vi "PKG_IMC_MoveAbs.vi"(4 "axis":i32, 5 "wait":i32, 6 "tgvel":dbl, 7 "endvel":dbl, 9 "startvel":dbl, 10 "pos":i32, 11 "handle":u32) -> (2 "function return":i32, 3 "handle out":u32)   [LabVIEW 2018, in "IMC_Pkg4xxx.lvlib"]
doc: "PKG_IMC_MoveAbs(IMC_HANDLE handle, long pos, double startvel, double endvel, double tgvel, int wait, int axis);"
uses:
  IMC_Pkg4xxx.lvlib
  IMC_Pkg4xxx.dll
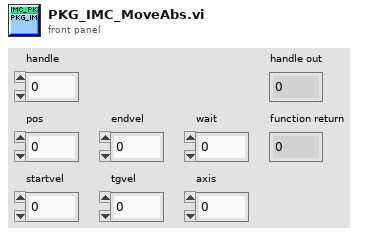
[diagram p1: front panel]
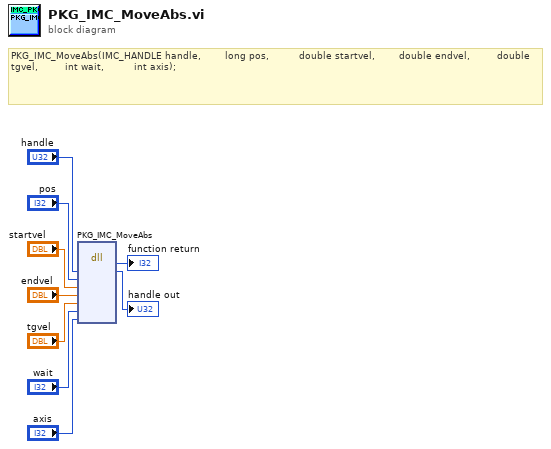
[diagram p0: block diagram]
diagram:
  # "PKG_IMC_MoveAbs(IMC_HANDLE handle, \t\t\t\t\t\t\tlong pos, \t\t\t\t\t\t\t\t\tdouble startvel, \t\t\t\t\t\t\tdouble endvel, \t\t\t\t\t\t\t\tdouble tgvel, \t\t\t\t\t\t\t\tint wait, \t\t\t\t\t\t\t\t\tint axis);"
  n1 = dll-call lib="PTH2\\abs D做的项目航天测量驱动电机IMCAppincLabview32\nIMC_Pkg4xxx.*" fn="PKG_IMC_MoveAbs"("handle"="handle", "pos"="pos", "startvel"="startvel", "endvel"="endvel", "tgvel"="tgvel", "wait"="wait", "axis"="axis") -> (→"function return":i32, "handle"=→"handle out":u32)  [unwired: 9 in, 2 out]
